vi "RUN ALL TESTS.vi"() -> ()   [LabVIEW 2013]
uses:
  <vilib>/addons/_JKI Toolkits/Caraya/classes/Test/Test.lvclass
panel:
  out "error out":errorcluster
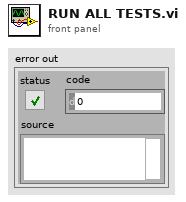
[diagram p1: front panel]
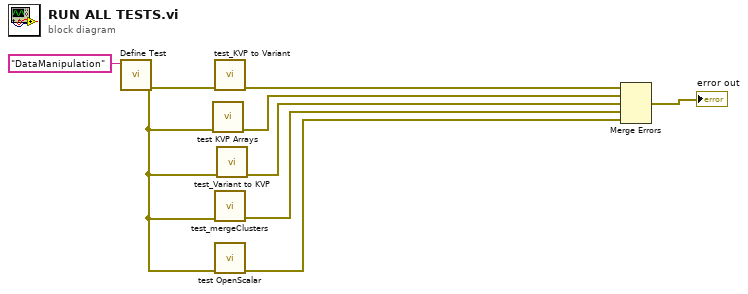
[diagram p0: block diagram]
diagram:
  n1 = call <vilib>:"Define Test.vi"("Label (VI Title)"="DataManipulation") -> ("error out"=w2:errorcluster)  [unwired: 10 in]
  n2 = call "test KVP Arrays.vi"("error in (no error)"=w2) -> ("error out"=w6:errorcluster)  [unwired: 10 in]
  n3 = call "test_KVP to Variant.vi"("error in (no error)"=w2) -> ("error out"=w7:errorcluster)  [unwired: 10 in]
  n4 = call "test_mergeClusters.vi"("error in (no error)"=w2) -> ("error out"=w4:errorcluster)  [unwired: 10 in]
  n5 = call "test OpenScalar.vi"("error in (no error)"=w2) -> ("error out"=w1:errorcluster)  [unwired: 10 in]
  n6 = call "test_Variant to KVP.vi"("error in (no error)"=w2) -> ("error out"=w5:errorcluster)  [unwired: 10 in]
  n7 = Merge Errors(w7, w6, w5, w4, w1) -> (→"error out":errorcluster)
